vi "Main.vi"(8 "error in (no error)":errorcluster, 11 "Application in":refnum<class "Application.lvclass">) -> (0 "error out":errorcluster, 3 "Application out":refnum<class "Application.lvclass">)   [LabVIEW 2018, in "Application.lvclass"]
doc: "Run this VI to lauch the State Machine."
uses:
  Application.lvclass
  Context/Context.lvclass
panel:
  # "Run this VI to lauch the State Machine."
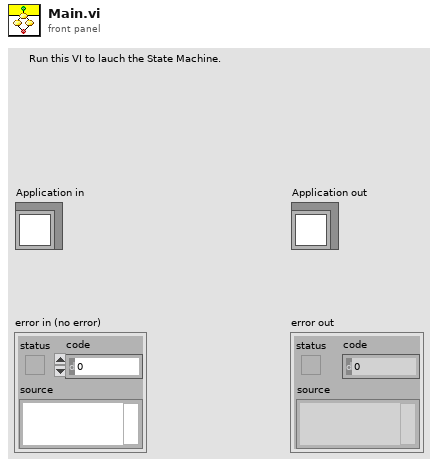
[diagram p1: front panel]
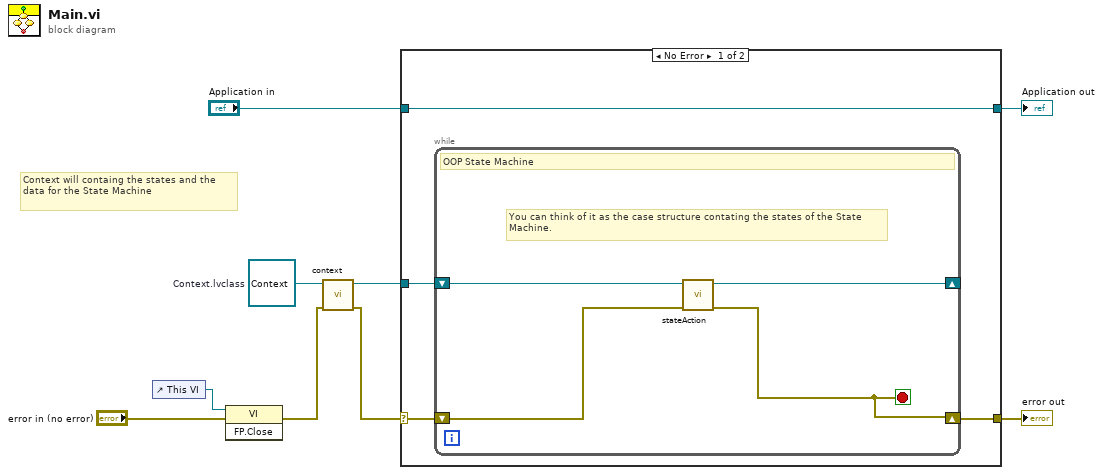
[diagram p0: block diagram]
diagram:
  w6 = refnum<class "Context.lvclass"> refnum  # Context.lvclass
  # "Context will containg the states and the\ndata for the State Machine"
  n1 = control-ref of="This VI"() -> (w1:refnum<vi>)
  n2 = invoke class="VI" method="FP.Close"(reference=w1, error in="error in (no error)") -> (error out=w2:errorcluster)  [unwired: 1 in, 2 out]
  n3 = call "context.vi"("error in (no error)"=w2, "Context in"=w6) -> ("error out"=w3:errorcluster, "Context out"=w5:refnum<class "Context.lvclass">)  [unwired: 8 in]
  n4 = case shown="No Error" w3 {
    selector: w3 -> [w12 w19]
    tunnel: [w11 w19] -> w9
    tunnel: [w13 w18] -> w7
    tunnel: "Application in" -> [w13 w18]
    tunnel: w5 -> [w10 _]
    frame No Error {
      n5 = while {
        shift-right: [w14] -> w11
        shift-left: w12 -> [w17]
        shift-right: [w15] -> _
        shift-left: w10 -> [w16]
        stop <- w14 stop-if-true
        # "You can think of it as the case structure contating the states of the State\nMachine."
        # "OOP State Machine"
        n6 = call "stateAction.vi"("error in (no error)"=w17, "Context in"=w16) -> ("error out"=w14:errorcluster, "Context out"=w15:refnum<class "Context.lvclass">)  [unwired: 8 in]
      }
    }
    frame Error {
    }
  }
  "error out" <- w9
  "Application out" <- w7
